vi "HFRR ADV v033 new software.vi"() -> ()   [LabVIEW 2025] (continued)
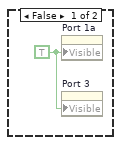
[diagram p5: hidden frame]
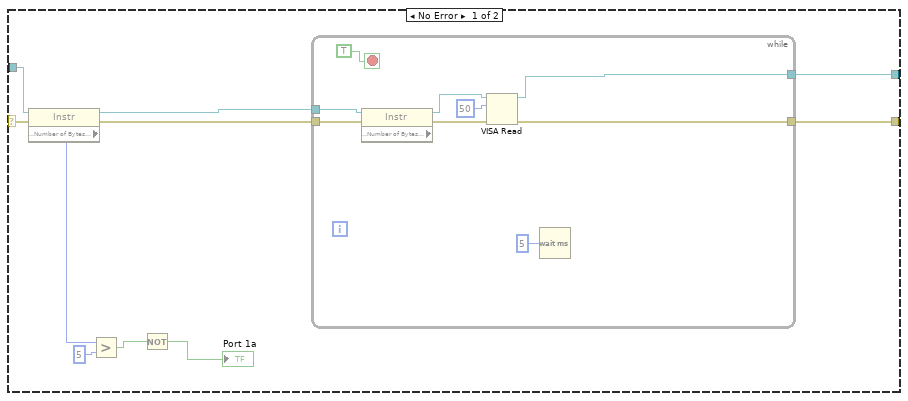
[diagram p6: hidden frame]
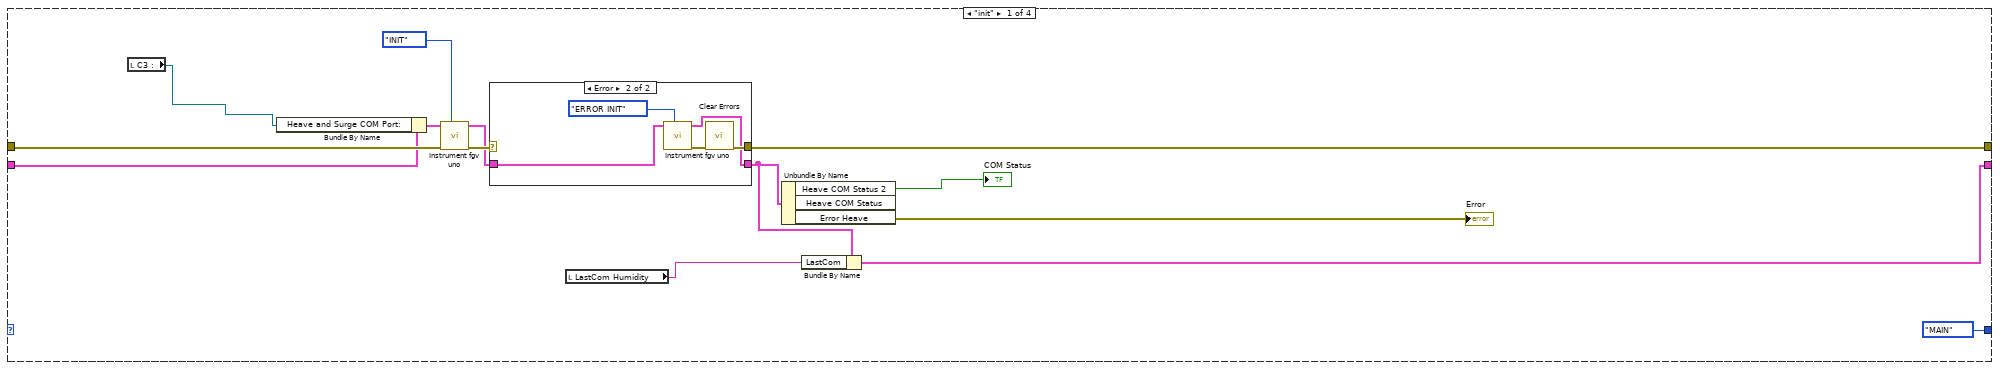
[diagram p8: hidden frame]
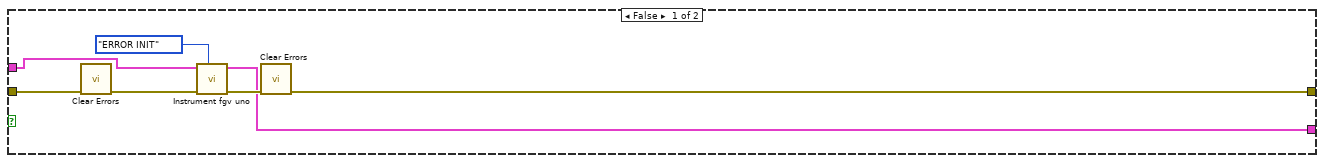
[diagram p10: hidden frame]
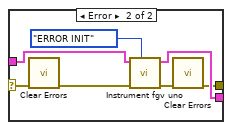
[diagram p12: hidden frame]
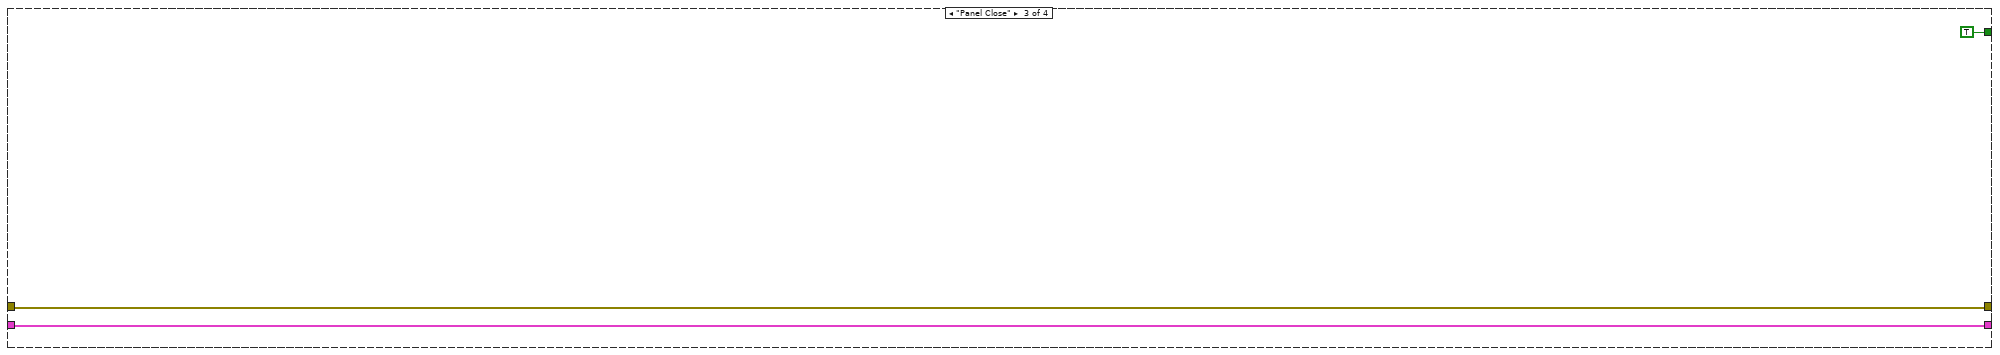
[diagram p14: hidden frame]
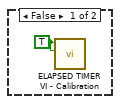
[diagram p18: hidden frame]
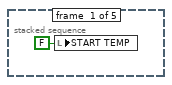
[diagram p20: hidden frame]
        n3356 = Select(t=enum16{"init", "MAIN", "Panel Close"}."Panel Close", s=w4334, f=enum16{"init", "MAIN", "Panel Close"}."MAIN") -> (s? t:f=w4333:enum16{"init", "MAIN", "Panel Close"})
      }
      frame "Panel Close" {
      }
      frame Default {
      }
    }
  }
  n3357 = while {
    shift-right: [w4402] -> _
    shift-left: _ -> [w4403]
    shift-right: [w4400] -> _
    shift-left: T20 {"Read Uno"="", "Bytes at Heave Port"=0.0, "UNO COM Port:"="COM9", "UNO COM Port: 2"="COM7", "Residual Due"="", "UNO COM Status 2"=TRUE, "UNO COM Status"=TRUE, "Port 2"=TRUE, "Sway PPR"=6400.0, "Surge PPR"=6400.0, "Heave PPR"=6400.0, "Sway Pitch"=2.0, "Surge Pitch"=3.0, "Heave Pitch"=4.0, "Sway Pulses/mm"=320.0, "Surge Pulses/mm"=1600.0, "Heave Pulses/mm"=1600.0, "inner loop"=0.0, "Read Heave and Surge 2"="", "String 36"="", "Write S"=FALSE, "WriteCC1"=[""], "Heave COM Loop"=0, "LastCom"="", "EXIT"=FALSE, "Error Heave"={"status"=TRUE, "code"=-1073807343, "source"=""}} -> [w4399]
    shift-right: [w4397] -> _
    shift-left: enum16{"init", "MAIN", "Panel Close"}."init" -> [w4398]
    stop <- w4401 stop-if-true
    # "UNO CODE LOGIC"
    n3358 = case shown="\"MAIN\"" w4398 {
      tunnel: w4403 -> [w4417 w4436 w4492 w4494]
      tunnel: [w4412 w4441 w4492 w4494] -> w4402
      tunnel: [_ _ TRUE _] -> w4401
      tunnel: [w4408 w4439 w4490 w4493] -> w4400
      tunnel: w4399 -> [w4414 w4435 w4490 w4493]
      tunnel: [enum16{"init", "MAIN", "Panel Close"}."MAIN" w4430 _ _] -> w4397
      frame "init" {
        n3359 = local read "Com Port 1"() -> (w4404:refnum<visa-resource-name>)
        n3360 = Bundle By Name(cluster=w4414, "UNO COM Port:"=w4404) -> (w4413:T20)
        n3361 = call "Instrument fgv.vi"("Enum"=T31."INIT", "error in (no error) 2"=w4417, "INPUT"=w4413) -> ("error"=w4415:errorcluster, "output"=w4411:T18)  [unwired: 6 in, 1 out]
        n3362 = case shown="Error" w4415 {
          selector: w4415 -> [w4419 _]
          tunnel: [w4419 w4423] -> w4412
          tunnel: w4411 -> [w4418 w4421]
          tunnel: [w4418 w4420] -> w4409
          frame No Error {
          }
          frame Error {
            n3363 = call "Instrument fgv.vi"("Enum"=T31."ERROR INIT", "INPUT"=w4421) -> ("error"=w4424:errorcluster, "output"=w4420:T18)  [unwired: 7 in, 1 out]
            n3364 = call <vilib>:"Clear Errors.vi"("error in (no error)"=w4424) -> ("error out"=w4423:errorcluster)  [unwired: 5 in, 1 out]
          }
        }
        n3365 = local read "LastCom UNO"() -> (w4406:string)
        n3366 = Unbundle By Name(w4409) -> ("Heave COM Status 2"=→"Instrument Status":bool, "Error Heave"=→"Error  2":errorcluster)  [unwired: 1 out]
        n3367 = Bundle By Name(cluster=w4409, "LastCom"=w4406) -> (w4408:T18)
      }
      frame "MAIN" {
        n3368 = Unbundle By Name(w4435) -> ("UNO COM Port: 2"=w4425:refnum<visa-resource-name>)
        n3369 = local read "Com Port 1"() -> (w4426:refnum<visa-resource-name>)
        n3370 = local write "COM Port UNO :"(w4425) -> ()
        n3371 = Equal?(x=w4425, y=w4426) -> (x = y?=w4442:bool)
        n3372 = Bundle By Name(cluster=w4435, "UNO COM Port:"=w4426) -> (w4434:T20)
        n3373 = case shown="True" w4442 {
          tunnel: [w4446 w4463] -> w4441
          tunnel: w4436 -> [w4447 w4469]
          tunnel: w4434 -> [w4445 w4467]
          tunnel: [w4444 w4462] -> w4439
          frame False {
            n3374 = call <vilib>:"Clear Errors.vi"("error in (no error)"=w4447) -> ("error out"=w4443:errorcluster)  [unwired: 5 in, 1 out]
            n3375 = call "Instrument fgv.vi"("Enum"=T31."ERROR INIT", "error in (no error) 2"=w4443, "INPUT"=w4445) -> ("error"=w4449:errorcluster, "output"=w4444:T18)  [unwired: 6 in, 1 out]
            n3376 = call <vilib>:"Clear Errors.vi"("error in (no error)"=w4449) -> ("error out"=w4446:errorcluster)  [unwired: 5 in, 1 out]
          }
          frame True {
            n3377 = call "Instrument fgv.vi"("Enum"=T31."READ", "error in (no error) 2"=w4469, "INPUT"=w4467) -> ("error"=w4468:errorcluster, "output"=w4461:T18)  [unwired: 6 in, 1 out]
            n3378 = Bundle By Name(cluster=w4461, "String 36"="WRITE UNO") -> (w4460:T18)
            n3379 = case shown="True" "Write" {
              selector: "Write" -> [_ w4484]
              tunnel: w4468 -> [w4482 w4489]
              tunnel: [w4482 w4488] -> w4458
              tunnel: w4460 -> [w4481 w4486]
              tunnel: [w4481 w4485] -> w4457
              frame False {
              }
              frame True {
                n3380 = Not(x=w4484) -> (.not. x?=w4483:bool)
                n3381 = local write "Write"(w4483) -> ()
                n3382 = call "Instrument fgv.vi"("Enum"=T31."MANUAL WRITE", "error in (no error) 2"=w4489, "INPUT"=w4486) -> ("error"=w4488:errorcluster, "output"=w4485:T18)  [unwired: 6 in, 1 out]
              }
            }
            n3383 = Array Size(array="Write UNO") -> (size(s)=w4455:i32)
            n3384 = Greater Than 0?(x=w4455) -> (x > 0?=w4454:bool)
            n3385 = call "Instrument fgv.vi"("Enum"=T31."WRITE", "error in (no error) 2"=w4458, "WriteCC1"="Write UNO", "INPUT"=w4457) -> ("error"=w4465:errorcluster, "WriteCC1 2"=w4456:string[], "output"=w4464:T18)  [unwired: 5 in]
            n3386 = case shown="True" w4454 {
              tunnel: w4456 -> [_ w4471]
              frame False {
              }
              frame True {
                n3387 = local write "Write UNO"(w4471) -> ()
              }
            }
            n3388 = case shown="Error" w4465 {
              selector: w4465 -> [w4472 w4475]
              tunnel: w4464 -> [w4473 w4480]
              tunnel: [w4473 w4479] -> w4462
              tunnel: [w4472 w4477] -> w4463
              frame No Error {
              }
              frame Error {
                n3389 = call <vilib>:"Clear Errors.vi"("error in (no error)"=w4475) -> ("error out"=w4474:errorcluster)  [unwired: 5 in, 1 out]
                n3390 = call "Instrument fgv.vi"("Enum"=T31."ERROR INIT", "error in (no error) 2"=w4474, "INPUT"=w4480) -> ("error"=w4478:errorcluster, "output"=w4479:T18)  [unwired: 6 in, 1 out]
                n3391 = call <vilib>:"Clear Errors.vi"("error in (no error)"=w4478) -> ("error out"=w4477:errorcluster)  [unwired: 5 in, 1 out]
              }
            }
            n3392 = Unbundle By Name(w4462) -> ("LastCom"=→"LastCom UNO":string, "Read Heave and Surge"=→"Read UNO":string)
          }
        }
        n3393 = Unbundle By Name(w4439) -> ("Heave COM Status 2"=w4440:bool, "Heave COM Status"=w4429:bool, "Error Heave"=w4427:errorcluster, "Bytes at Heave Port"=→"Bytes at Humidity Port":dbl)
        n3394 = Not(x=w4429) -> (.not. x?=w4437:bool)
        n3395 = Not(x=w4440) -> (.not. x?=w4428:bool)
        n3396 = local write "Instrument Status"(w4437) -> ()
        n3397 = local write "Error  2"(w4427) -> ()
        n3398 = local write "Port 1a"(w4429) -> ()
        n3399 = local read "Quit"() -> (w4431:bool)
        n3400 = local write "COM Status"(w4428) -> ()
        n3401 = Select(t=enum16{"init", "MAIN", "Panel Close"}."Panel Close", s=w4431, f=enum16{"init", "MAIN", "Panel Close"}."MAIN") -> (s? t:f=w4430:enum16{"init", "MAIN", "Panel Close"})
      }
      frame "Panel Close" {
      }
      frame Default {
      }
    }
  }
  n3402 = while {
    stop <- w4520 stop-if-true
    n3403 = local read "Read HUMIDITY"() -> (w4495:string)
    n3404 = call <vilib>:"High Resolution Polling Wait.vi"("seconds to wait"=0.05) -> ()  [unwired: 10 in, 1 out]
    n3405 = Spreadsheet String To Array(delimiter (Tab)=",", format string="", spreadsheet string=w4495, array type (2D Dbl)=string[] []) -> (array=w4515:string[])
    n3406 = for {
      tunnel: w4515 -> [w4525] mode=indexing
      tunnel: string[] ["STATE;", "SET;", "RH;", "T;", "AMB_RH;", "AMB_T;", "PUMP;", "FAN_IN;", "FAN_OUT;", "DEHUM;", "CURRENT;", "STALL;"] -> [w4524] mode=indexing
      tunnel: [w4523] -> w4514 mode=indexing
      n3407 = Match Pattern(string=w4525, regular expression=w4524) -> (after substring=w4523:string)  [unwired: 1 in, 3 out]
    }
    n3408 = Index Array(array=w4514) -> (element #1=→"STATE :":string, element #2=→"SET :":string, element #3=w4503:string, element #4=→"T :":string, element #5=w4501:string, element #6=→"AMB_T :":string, element #7=→"PUMP :":string, element #8=→"FAN_IN :":string, element #9=→"FAN_OUT :":string, element #10=→"DEHUM :":string, element #11=→"CURRENT :":string, element #12=→"STALL :":string)  [unwired: 12 in]
    "RH :" <- w4503
    "AMB_RH :" <- w4501
    n3409 = Fract/Exp String To Number(string=w4503) -> (number=w4496:dbl)  [unwired: 3 in, 1 out]
    n3410 = Fract/Exp String To Number(string=w4501) -> (number=w4500:dbl)  [unwired: 3 in, 1 out]
    n3411 = local write "Ambient Humidity :"(w4500) -> ()
    n3412 = Equal?(x=w4496, y=0.0) -> (x = y?=w4498:bool)
    n3413 = case shown="True" w4498 {
      tunnel: [w4521 w4522] -> w4497
      tunnel: w4496 -> [w4521 _]
      frame False {
        (unwired) 0.0
        "Humidity temp" <- w4521
      }
      frame True {
        n3414 = local read "Humidity temp"() -> (w4522:dbl)
      }
    }
    "RH Numeric:" <- w4497
    n3415 = local read "Quit"() -> (w4520:bool)
  }
